vi "initialise.vi"(8 "error in (no error)":errorcluster, 11 "GenericPlugin in":refnum<class "FPGAWrapperDL090211Galvo.lvclass">) -> (0 "error out":errorcluster, 3 "GenericPlugin out":refnum<class "FPGAWrapperDL090211Galvo.lvclass">)   [LabVIEW 2010, in "FPGAWrapperDL090211Galvo.lvclass"]
doc: "The dynamic dispatch-version of this VI initalises the plug-in object by allocating and initalising any dynamic resources need."
uses:
  FPGAWrapperDL090211Galvo.lvclass
  GenericFPGAWrapper/GenericFPGAWrapper/GenericFPGAWrapper.lvclass
  <vilib>/userDefined/High Color/nirio_resource_hc.ctl
  config_data_cluster.ctl
  bit_file_enum.ctl
  common_typedefs/pixel_to_host_enum.ctl
  <vilib>/rvi/interface/nirviOpenFPGA/nirviOpenFPGA.xnode
  FPGA Bitfiles/FPGAWrapperDL090211_PXI-7813R_80MHz.lvbitx
  <vilib>/rvi/ClientSDK/nirviWhatTheDeviceIsDoing.ctl
  FPGA Bitfiles/FPGAWrapperDL090211_PXI-7813R_120MHz.lvbitx
  <vilib>/rvi/interface/nirviMethod/nirviMethod.xnode
  <vilib>/rvi/interface/nirviReadWriteControl/nirviReadWriteControl.xnode
  <vilib>/rvi/interface/common/niFpgaNodeNameForErrorReporting.ctl
  <vilib>/rvi/errors/niLvFpgaWhatHappensToTopLevelVI.ctl
  <vilib>/FPGAPlugInAG/PXI-7813R/niLvFpga_Open_PXI-7813R.vi
  <vilib>/rvi/interface/common/dynamic/niFpgaDynamicAddResources.vi
  <vilib>/FPGAPlugInAG/Dynamic/niLvFpga_Reset_Dynamic.vi
  <vilib>/Utility/error.llb/Error Cluster From Error Code.vi
  <vilib>/rvi/errors/niLvFpgaAdjustHostInterfaceError.vi
  NiFpgaLv.dll
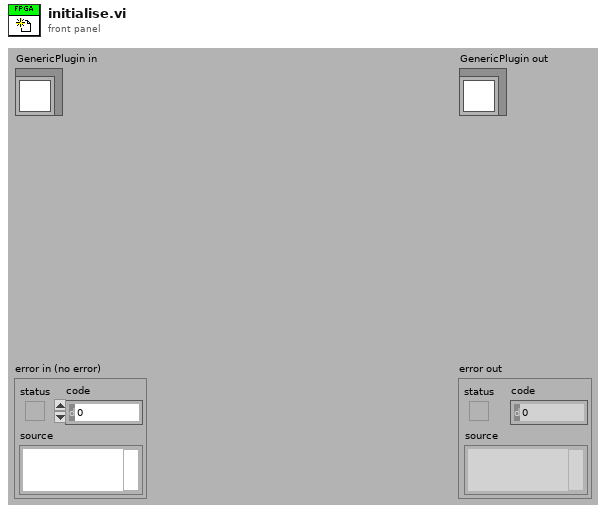
[diagram p1: front panel]
types:
  T1 = typedef "nirio_resource_hc.ctl" = tag
  T2 = typedef "FPGAWrapperDL090211Galvo.lvclass/config_data_cluster.ctl" = cluster{"bit file":T3, "hifo box version":i32, "ADC clock phase":i32, "pixel-to-host mode":T4}
  T3 = typedef "FPGAWrapperDL090211Galvo.lvclass/bit_file_enum.ctl" = enum16{"80MHz for PXI-7813R", "120MHz for PXI-7813R"}
  T4 = typedef "pixel_to_host_enum.ctl" = enum16{"3-channel mode", "4-channel mode"}
  T5 = typedef "nirviWhatTheDeviceIsDoing.ctl" = enum32{"nothing", "something other than LabVIEW FPGA", "FPGA interface", "interactive", "emulation"}
  T6 = typedef "niFpgaNodeNameForErrorReporting.ctl" = enum16{"Open FPGA VI Reference", "Read/Write Control", "Invoke Method: Abort", "Invoke Method: Acknowledge IRQ", "Invoke Method: Download", "Invoke Method: FIFO.Configure", "Invoke Method: FIFO.Read", "Invoke Method: FIFO.Start", "Invoke Method: FIFO.Stop", "Invoke Method: FIFO.Write", "Invoke Method: Reset", "Invoke Method: Run", "Invoke Method: Wait on IRQ", "Close FPGA VI Reference"}
  T7 = typedef "niLvFpgaWhatHappensToTopLevelVI.ctl" = enum16{"top level VI scripted behind XNode", "top level VI inlined behind XNode"}
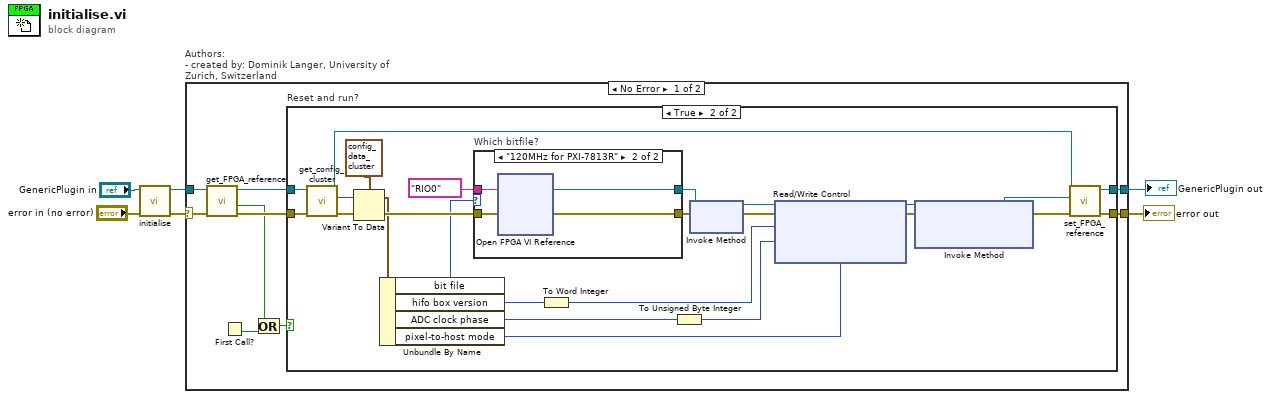
[diagram p0: block diagram]
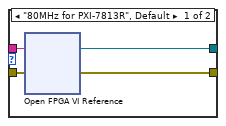
[diagram p3: hidden frame]
diagram:
  n1 = call-parent "initialise.vi"("error in (no error)"="error in (no error)", "GenericPlugin in"="GenericPlugin in") -> ("error out"=w4:errorcluster, "GenericPlugin out"=w3:refnum<class "FPGAWrapperDL090211Galvo.lvclass">)  [unwired: 8 in]
  n2 = case "Authors: \n- created by: Dominik Langer, University of Zurich, Switzerland" shown="No Error" w4 {
    selector: w4 -> [w15 w246]
    tunnel: w3 -> [w13 w247]
    tunnel: [w8 w246] -> w2
    tunnel: [w7 w247] -> w1
    frame No Error {
      n3 = call-dynamic "get_FPGA_reference.vi"("error in (no error)"=w15, "FPGAWrapperDL090211Galvo in"=w13) -> ("error out"=w14:errorcluster, "is empty?"=w11:bool, "FPGAWrapperDL090211Galvo out"=w9:refnum<class "FPGAWrapperDL090211Galvo.lvclass">)  [unwired: 6 in, 1 out]
      n4 = First Call?() -> (First Call?: T/F=w12:bool)
      n5 = Or(x=w11, y=w12) -> (x .or. y?=w10:bool)
      n6 = case "Reset and run?" shown="True" w10 {
        tunnel: w14 -> [w16 w42]
        tunnel: w9 -> [w17 w41]
        tunnel: [w16 w32] -> w8
        tunnel: [w17 w31] -> w7
        frame False {
        }
        frame True {
          n7 = call-dynamic "get_config_cluster.vi"("error in (no error)"=w42, "FPGAWrapperDL090211Galvo in"=w41) -> ("error out"=w40:errorcluster, "config cluster (variant)"=w38:variant, "FPGAWrapperDL090211Galvo out"=w28:refnum<class "FPGAWrapperDL090211Galvo.lvclass">)  [unwired: 7 in]
          n8 = Variant To Data(error in=w40, Variant=w38, type=T2 {"bit file"=enum."80MHz for PXI-7813R", "hifo box version"=0, "ADC clock phase"=0, "pixel-to-host mode"=enum."3-channel mode"} ("config data")) -> (error out=w39:errorcluster, data=w36:T2)
          n9 = Unbundle By Name(w36) -> ("bit file"=w21:T3, "hifo box version"=w25:i32, "ADC clock phase"=w27:i32, "pixel-to-host mode"=w20:T4)
          n10 = case "Which bitfile?" shown="\"120MHz for PXI-7813R\"" w21 {
            tunnel: w39 -> [w46 w65]
            tunnel: [w45 w63] -> w35
            tunnel: T1 "RIO0" ("resource name") -> [w44 w64]
            tunnel: [w43 w62] -> w18
            frame "80MHz for PXI-7813R", Default {
              n11 = xnode "Open FPGA VI Reference"("error in"=w46, "resource name"=w44) -> ("FPGA VI Reference Out"=w43:refnum<k20>, "error out"=w45:errorcluster)
            }
            frame "120MHz for PXI-7813R" {
              n12 = xnode "Open FPGA VI Reference"("error in"=w65, "resource name"=w64) -> ("FPGA VI Reference Out"=w62:refnum<k20>, "error out"=w63:errorcluster)
            }
          }
          n13 = To Word Integer(number=w25) -> (16bit integer=w24:i16)
          n14 = To Unsigned Byte Integer(number=w27) -> (unsigned 8bit integer=w26:u8)
          n15 = xnode "Invoke Method"("FPGA VI Reference In"=w18, "error in"=w35) -> ("FPGA VI Reference Out"=w19:refnum<k20>, "error out"=w29:errorcluster)
          n16 = xnode "Read/Write Control"("FPGA VI Reference In"=w19, "error in"=w29, "converter box version"=w24, "ADC clock phase"=w26, "pixel-to-host mode"=w20) -> ("FPGA VI Reference Out"=w34:refnum<k20>, "error out"=w30:errorcluster)
          n17 = xnode "Invoke Method"("FPGA VI Reference In"=w34, "error in"=w30) -> ("FPGA VI Reference Out"=w23:refnum<k20>, "error out"=w33:errorcluster)  [unwired: 1 in]
          n18 = call-dynamic "set_FPGA_reference.vi"("error in (no error)"=w33, "FPGA VI reference"=w23, "FPGAWrapperDL090211Galvo in"=w28) -> ("error out"=w32:errorcluster, "FPGAWrapperDL090211Galvo out"=w31:refnum<class "FPGAWrapperDL090211Galvo.lvclass">)  [unwired: 7 in]
        }
      }
    }
    frame Error {
    }
  }
  "error out" <- w2
  "GenericPlugin out" <- w1
